vi "UI.vi"(8 "error in (no error)":errorcluster, 11 "Multiply in":refnum<class "Multiply.lvclass">) -> (0 "error out":errorcluster, 3 "Multiply out":refnum<class "Multiply.lvclass">)   [LabVIEW 2020, in "Multiply.lvclass"]
uses:
  Multiply.lvclass
  C:/Users/Khishore/Downloads/Assignment 25 3/Assignment 25/Arithmetic Operations/Arithmetic Operations.lvclass
  Typedefs/User event operations.ctl
  Arithmetic Operations.lvclass/Arithmetic Operations.ctl
  Accessors/Write/Write A.vi
  Accessors/Write/Write B.vi
  Accessors/Read/Read C.vi
  Accessors/Read/Read A.vi
  Accessors/Read/Read B.vi
  Simple calculator.lvlib
panel:
  out "C":dbl
  in  "B":dbl
  in  "A":dbl
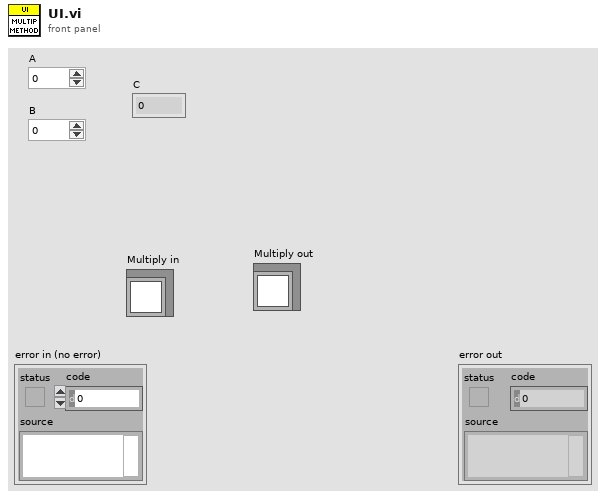
[diagram p1: front panel]
types:
  T1 = typedef "Simple calculator.lvlib/User event operations.ctl" = enum16{"Create", "Get Ref", "Generate ", "Destroy"}
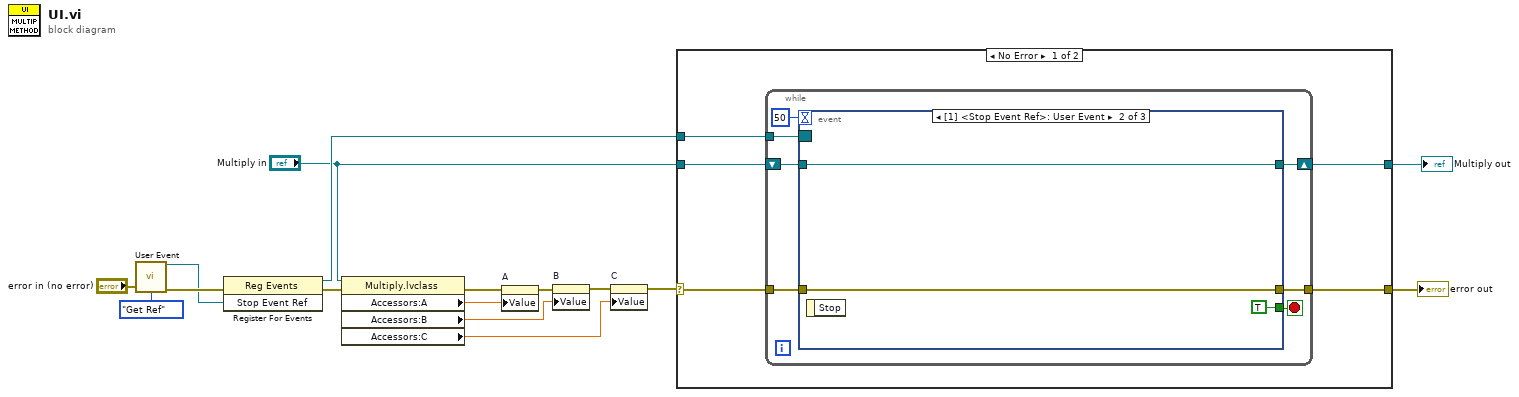
[diagram p0: block diagram]
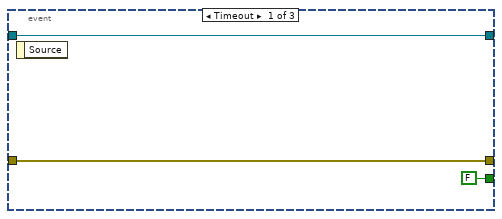
[diagram p2: hidden frame]
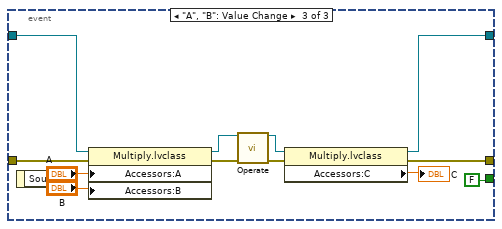
[diagram p3: hidden frame]
diagram:
  n1 = call "User Event.vi"("Error in"="error in (no error)", "Operation"=User_event_operations."Get Ref") -> ("Stop Event Ref"=w13:refnum<user-event>, "Error out"=w14:errorcluster)  [unwired: 12 in]
  n2 = register-events(error in=w14, w13) -> (reference out=w11:refnum<event-registration>, error out=w10:errorcluster)  [unwired: 1 in]
  n3 = property class="Multiply.lvclass"(reference="Multiply in", error in=w10) -> (error out=w8:errorcluster, "Accessors:A"=w4:dbl, "Accessors:B"=w3:dbl, "Accessors:C"=w2:dbl)  [unwired: 1 out]
  n4 = property on="A" class="DigNum (strict)"(error in=w8, "Value"=w4) -> (error out=w7:errorcluster)  [unwired: 1 in, 1 out]
  n5 = property on="B" class="DigNum (strict)"(error in=w7, "Value"=w3) -> (error out=w6:errorcluster)  [unwired: 1 in, 1 out]
  n6 = property on="C" class="DigNum (strict)"(error in=w6, "Value"=w2) -> (error out=w5:errorcluster)  [unwired: 1 in, 1 out]
  n7 = case shown="No Error" w5 {
    selector: w5 -> [w18 w48]
    tunnel: [w19 w48] -> w16
    tunnel: [w21 w47] -> w15
    tunnel: "Multiply in" -> [w20 w47]
    tunnel: w11 -> [w17 _]
    frame No Error {
      n8 = while {
        tunnel: [w24] -> w19
        tunnel: w18 -> [w23]
        tunnel: w17 -> [w27]
        shift-right: [w26] -> w21
        shift-left: w20 -> [w25]
        stop <- w22 stop-if-true
        n9 = event shown="[1] <Stop Event Ref>: User Event" {
          selector: w27 -> [_ _ _]
          dyn-events: _ -> [_ _ _]
          timeout: 50 -> [_ _ _]
          tunnel: [w31 w34 w37] -> w26
          tunnel: w25 -> [w31 w34 w45]
          tunnel: [w30 w33 w38] -> w24
          tunnel: w23 -> [w30 w33 w46]
          tunnel: [FALSE ("Stop") TRUE ("Stop") FALSE ("Stop")] -> w22
          event Timeout {
            n10 = event-data() -> ()  [unwired: 1 in, 1 out]
          }
          event User Event {
            n11 = event-data() -> ()  [unwired: 1 in, 1 out]
          }
          event "A", "B": Value Change {
            n12 = event-data() -> ()  [unwired: 1 in, 1 out]
            n13 = property class="Multiply.lvclass"(reference=w45, error in=w46, "Accessors:A"="A", "Accessors:B"="B") -> (reference out=w41:refnum<class "Multiply.lvclass">, error out=w42:errorcluster)
            n14 = call-dynamic "Operate.vi"("Multiply in"=w41, "error in (no error)"=w42) -> ("Multiply out"=w36:refnum<class "Multiply.lvclass">, "error out"=w40:errorcluster)  [unwired: 12 in]
            n15 = property class="Multiply.lvclass"(reference=w36, error in=w40) -> (reference out=w37:refnum<class "Multiply.lvclass">, error out=w38:errorcluster, "Accessors:C"=→"C":dbl)
          }
        }
      }
    }
    frame Error {
    }
  }
  "error out" <- w16
  "Multiply out" <- w15
